vi "Create All Message Queues.vi"(8 "error in (no error)":errorcluster) -> (0 "error out":errorcluster, 3 "Message Queues out":T1)   [LabVIEW 2021, in "Message Queue.lvlib"]
doc: "This VI creates and initializes all the message queues for your application. If your application requires more than one message queue, right-click the \"Message Queues\" constant above and select Open Type Def. Add the new Message Queue(s) to the type definition, then initialize them in this VI."
uses:
  Message Queue.lvlib
  All Message Queues.ctl
  Message Cluster.ctl
  Enqueue Message (Single).vi
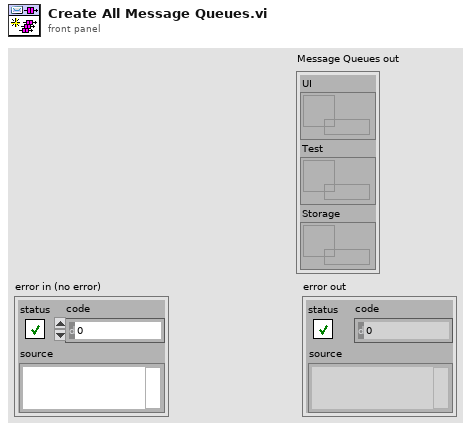
[diagram p1: front panel]
types:
  T1 = typedef "Message Queue.lvlib/All Message Queues.ctl" = cluster{"UI":refnum<queue>, "Test":refnum<queue>, "Storage":refnum<queue>}
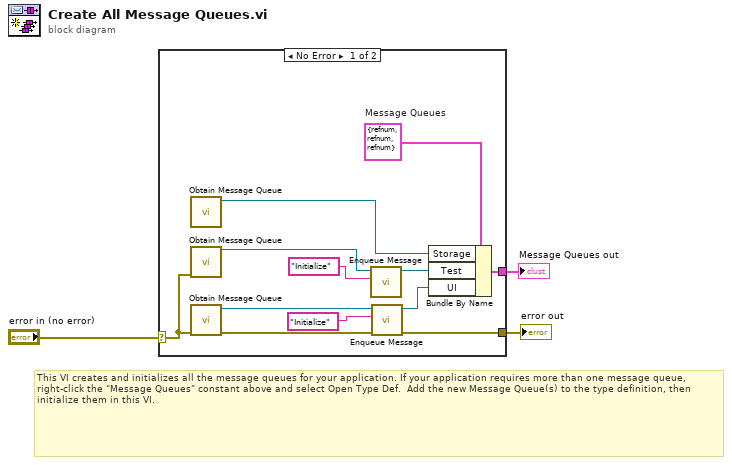
[diagram p0: block diagram]
diagram:
  # "This VI creates and initializes all the message queues for your application. If your application requires more than one message queue, right-click the \"Message Queues\" constant above and select Open Type Def.  Add the new Message Queue(s) to the type definition, then initialize them in this VI."
  n1 = case shown="No Error" "error in (no error)" {
    selector: "error in (no error)" -> [w9 w16]
    tunnel: [w15 w16] -> w3
    tunnel: [w13 _] -> w2
    frame No Error {
      w14 = T1 {"UI"=refnum, "Test"=refnum, "Storage"=refnum}  # Message Queues
      n2 = call "Obtain Message Queue.vi"() -> ("Message Queue UI"=w4:refnum<queue>)  [unwired: 10 in, 1 out]
      n3 = call "Obtain Message Queue.vi"("error in (no error)"=w9) -> ("Message Queue UI"=w6:refnum<queue>)  [unwired: 9 in, 1 out]
      n4 = call "Obtain Message Queue.vi"("error in (no error)"=w9) -> ("error out"=w12:errorcluster, "Message Queue UI"=w10:refnum<queue>)  [unwired: 9 in]
      n5 = call-poly "Enqueue Message.vi"("Message"="Initialize", "Message Queue"=w6) -> ("dup Message Queue"=w5:refnum<queue>)  [unwired: 8 in, 1 out]
      n6 = call-poly "Enqueue Message.vi"("error in (no error)"=w12, "Message"="Initialize", "Message Queue"=w10) -> ("error out"=w15:errorcluster, "dup Message Queue"=w8:refnum<queue>)  [unwired: 7 in]
      n7 = Bundle By Name(cluster=w14, "Storage"=w4, "Test"=w5, "UI"=w8) -> (w13:T1)
    }
    frame Error {
    }
  }
  "Message Queues out" <- w2
  "error out" <- w3
